vi "Screening.vi"(4 "Data type":T1 items=["AXON", "HEKA"], 5 "Screen threshold (dV/dt)":dbl=-5000.0 format="%#_13g", 6 "dt":dbl=0.0001 format="%#_13g", 7 "Detected Event (1D) In":cluster{dbl[][]}[](array[cluster]), 8 "Sweep trace (2D) In":cluster{"Ramp Pattern":dbl[], "X":dbl[]}[][](array[cluster])) -> (1 "Detected Event (1D) Out":cluster{dbl[][]}[](array[cluster]), 3 "Sweep trace (2D) Out":cluster{"Ramp Pattern":dbl[], "X":dbl[]}[][](array[cluster]))   [LabVIEW 2017]
uses:
  Data type_new.ctl
  <vilib>/Analysis/NI_AALPro.lvlib
panel:
  out "배열":bool[][](array[boolean])
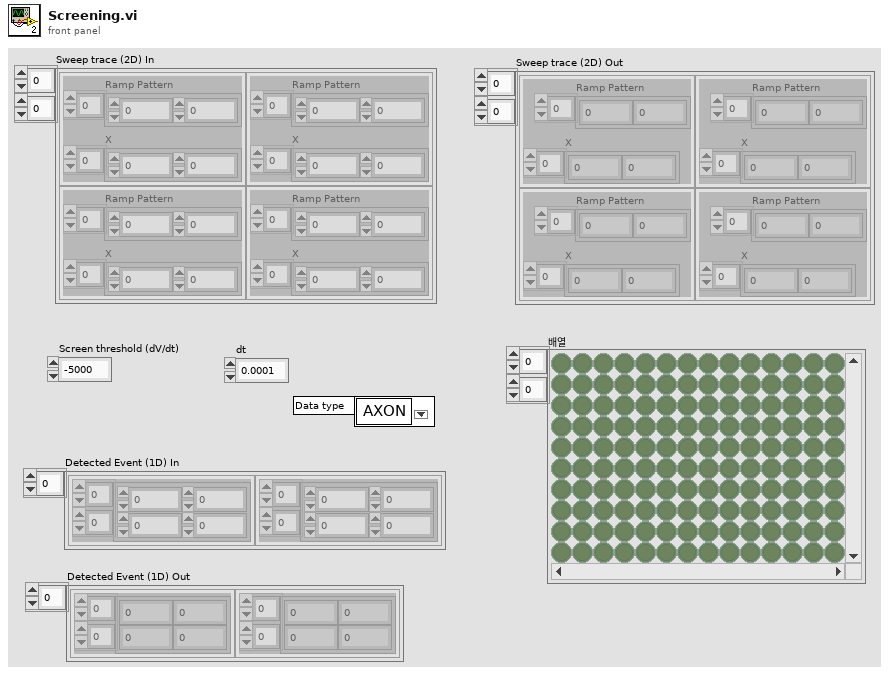
[diagram p1: front panel]
types:
  T1 = typedef "Data type_new.ctl" = u16
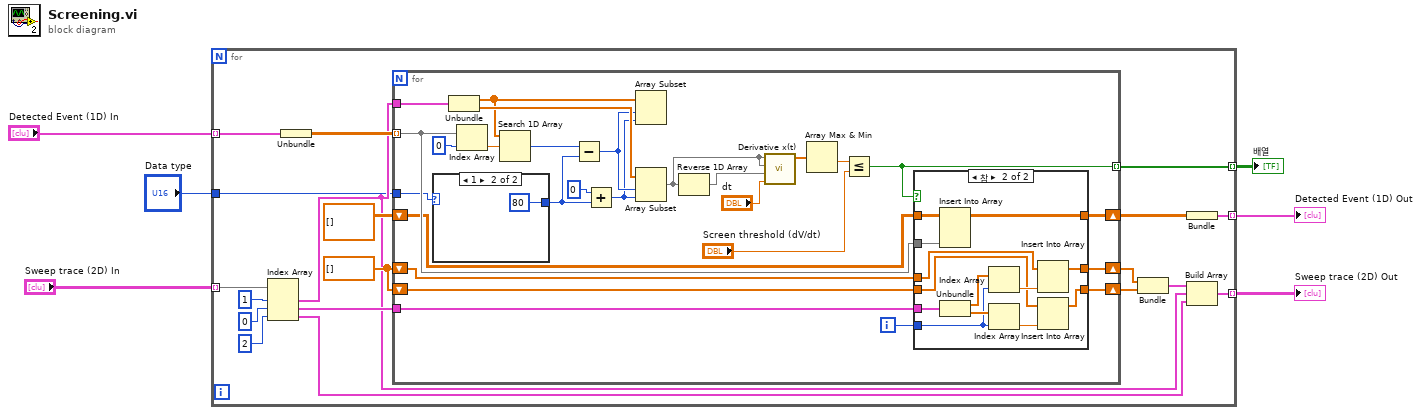
[diagram p0: block diagram]
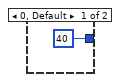
[diagram p2: hidden frame]
diagram:
  n1 = for {
    tunnel: "Sweep trace (2D) In" -> [w25] mode=indexing
    tunnel: "Detected Event (1D) In" -> [w23] mode=indexing
    tunnel: [w21] -> w5 mode=indexing
    tunnel: [w18] -> w4 mode=indexing
    tunnel: [w8] -> w3 mode=indexing
    tunnel: "Data type" -> [w7]
    w14 = dbl[] []
    n2 = Index Array(array=w25, index #1=1 ("인덱스"), index #2=0 ("인덱스"), index #3=2 ("인덱스")) -> (element #1=w10:cluster{"Ramp Pattern":dbl[], "X":dbl[]}, element #2=w16:cluster{"Ramp Pattern":dbl[], "X":dbl[]}, element #3=w9:cluster{"Ramp Pattern":dbl[], "X":dbl[]})
    n3 = Unbundle(w23) -> (w22:dbl[][])
    n4 = for {
      tunnel: w22 -> [w37] mode=indexing
      tunnel: w10 -> [w51]
      tunnel: [w39] -> w21 mode=indexing
      shift-right: [w36] -> w19
      shift-left: dbl[][] [] -> [w35]
      tunnel: w16 -> [w34]
      shift-right: [w32] -> w13
      shift-left: w14 -> [w31]
      shift-right: [w30] -> w12
      shift-left: w14 -> [w29]
      tunnel: w7 -> [w27]
      i -> [w33]
      n5 = case shown="1" w27 {
        tunnel: [40 ("y") 80 ("y")] -> w49
        frame 0, Default {
        }
        frame 1 {
        }
      }
      n6 = Unbundle(w51) -> ("Ramp Pattern"=w43:dbl[], "X"=w48:dbl[])
      n7 = Index Array(array=w37, index=0 ("인덱스")) -> (element=w38:dbl)
      n8 = Search 1D Array(1D array=w43, element=w38) -> (index of element=w26:i32)  [unwired: 1 in]
      n9 = Subtract(x=w26, y=w49) -> (x-y=w47:i32)
      n10 = Add(x=0, y=w49) -> (x+y=w46:i32)
      n11 = Array Subset(array=w43, index=w47, length=w46) -> ()  [unwired: 1 out]
      n12 = Array Subset(array=w48, index=w47, length=w46) -> (w42:dbl[])
      n13 = Reverse 1D Array(array=w42) -> (reversed array=w44:dbl[])
      n14 = call <vilib>:"Derivative x(t).vi"("dt"="dt", "Final Condition"=w44, "Initial Condition"=w42, "X"=w42) -> ("dX/dt"=w28:dbl[])  [unwired: 6 in, 1 out]
      n15 = Array Max & Min(array=w28) -> (min value=w41:dbl)  [unwired: 3 out]
      n16 = Less Or Equal?(x=w41, y="Screen threshold (dV/dt)") -> (x <= y?=w39:bool)
      n17 = case shown="참" w39 {
        tunnel: w37 -> [_ w70]
        tunnel: [w57 w69] -> w36
        tunnel: w35 -> [w57 w68]
        tunnel: w34 -> [_ w67]
        tunnel: w33 -> [_ w64]
        tunnel: [w55 w61] -> w32
        tunnel: w31 -> [w55 w60]
        tunnel: [w56 w59] -> w30
        tunnel: w29 -> [w56 w58]
        frame False {
        }
        frame True {
          n18 = Insert Into Array(array=w68, new element=w70) -> (w69:dbl[][])  [unwired: 2 in]
          n19 = Unbundle(w67) -> ("Ramp Pattern"=w66:dbl[], "X"=w65:dbl[])
          n20 = Index Array(array=w66, index=w64) -> (element=w63:dbl)
          n21 = Index Array(array=w65, index=w64) -> (element=w62:dbl)
          n22 = Insert Into Array(array=w58, new element=w63) -> (w59:dbl[])  [unwired: 1 in]
          n23 = Insert Into Array(array=w60, new element=w62) -> (w61:dbl[])  [unwired: 1 in]
        }
      }
    }
    n24 = Bundle(w12, w13) -> (w11:cluster{dbl[], dbl[]})  [unwired: 1 in]
    n25 = Bundle(w19) -> (w18:cluster{dbl[][]})  [unwired: 1 in]
    n26 = Build Array(w11, w10, w9) -> (w8:cluster{"Ramp Pattern":dbl[], "X":dbl[]}[])
  }
  "배열" <- w5
  "Detected Event (1D) Out" <- w4
  "Sweep trace (2D) Out" <- w3
